vi "Read Folder.vi"(8 "error in (no error)":errorcluster, 11 "Context in":T1) -> (0 "error out":errorcluster, 3 "Context out":T1)   [LabVIEW 2020, in "DocTool.lvlib"]
uses:
  DocTool.lvlib
  TDefs/Context.ctl
  Events.ctl
  UserEvent.ctl
  TDefs/State.ctl
  TDefs/States.ctl
  TDefs/Single File Properties.ctl
  TDefs/FP Items Properties.ctl
  TDefs/FP Item Properties.ctl
  TDefs/CopyTag.ctl
  StateMachine.lvlib
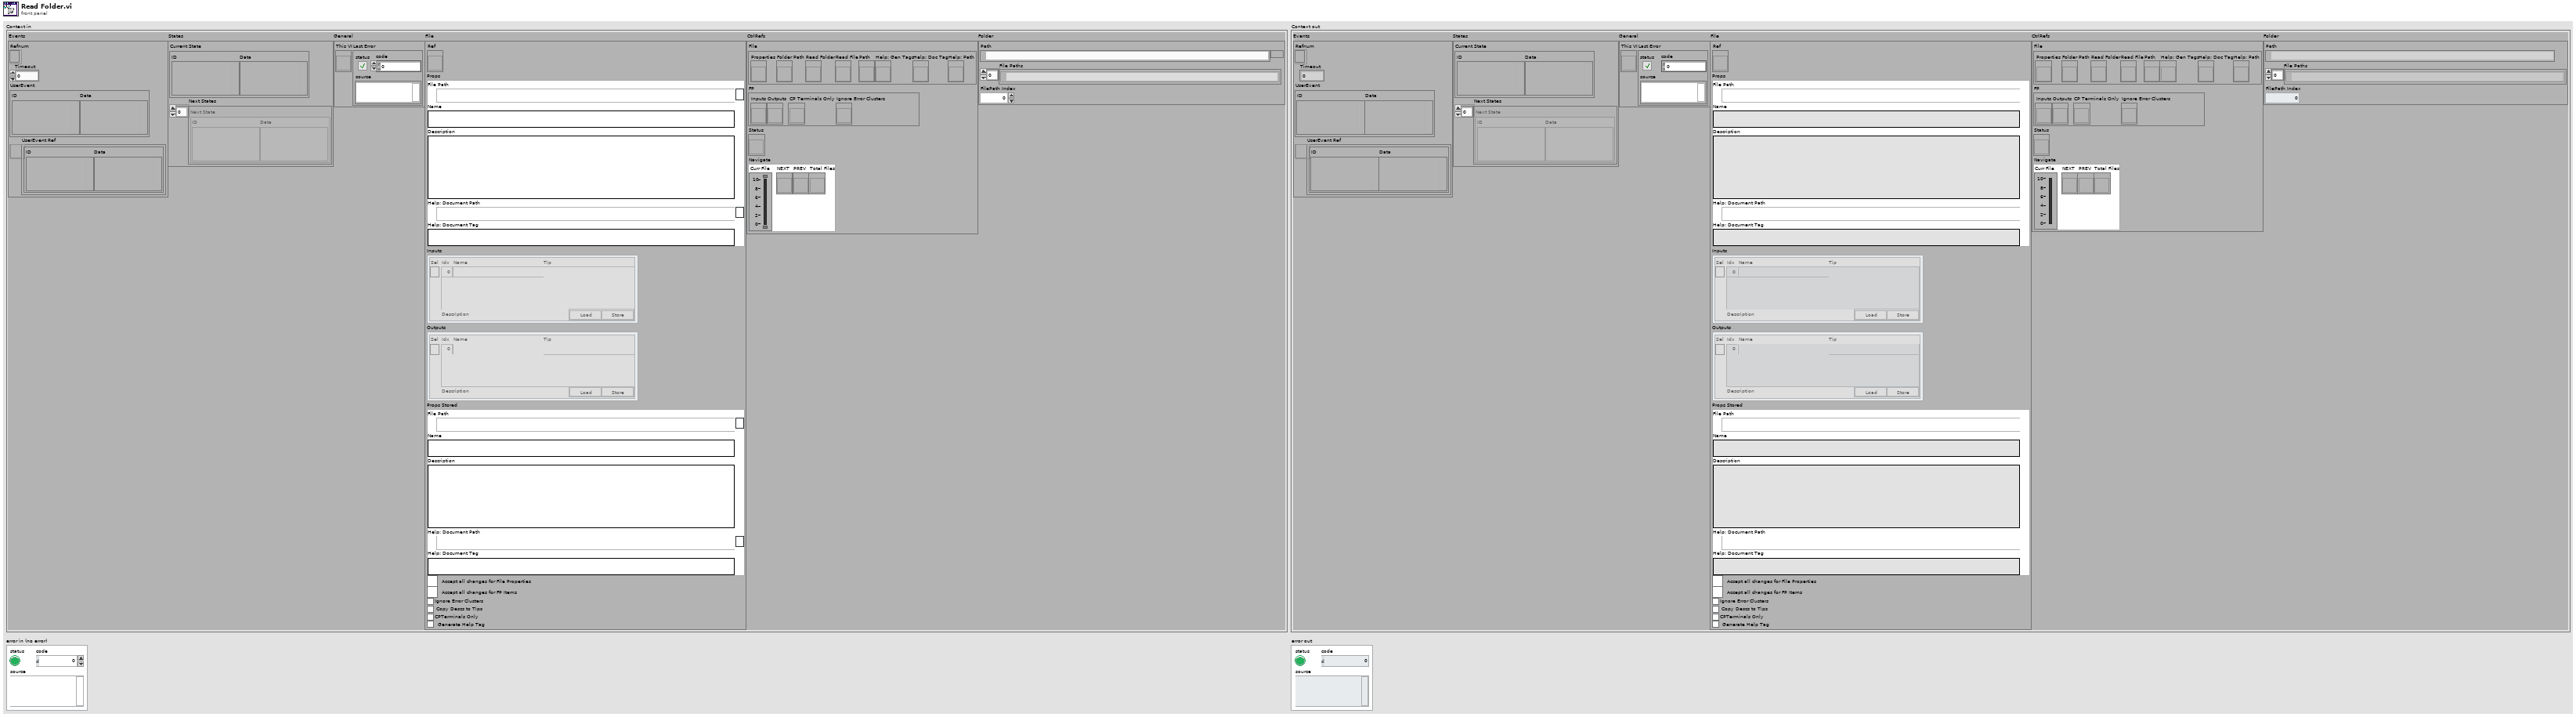
[diagram p1: front panel]
types:
  T1 = typedef "DocTool.lvlib/Context.ctl" = cluster{"Events":T2, "States":cluster{"Current State":T4, "Next States":T5}, "General":cluster{"This VI":refnum<vi>, "Last Error":errorcluster}, "File":cluster{"Ref":refnum<vi>, "Props":T6, "Inputs":T7, "Outputs":T7, "Props Stored":T6, "Write":bool, "Write FP":bool, "Ignore Error Clusters":bool, "Copy Descs to Tips":bool, "CPTerminals Only":bool, "Generate Help Tag":bool}, "CtrlRefs":cluster{"File":cluster{"Properties":refnum<vi>, "Folder Path":refnum<vi>, "Read Folder":refnum<vi>, "Read File":refnum<vi>, "Path":refnum<vi>, "Help: Gen Tags":refnum<vi>, "Help: Doc Tag":refnum<vi>, "Help: Path":refnum<vi>}, "FP":cluster{"Inputs":refnum<vi>, "Outputs":refnum<vi>, "CP Terminals Only":refnum<vi>, "Ignore Error Clusters":refnum<vi>}, "Status":refnum<vi>, "Navigate":cluster{"Curr File":refnum<vi>, "NEXT":refnum<vi>, "PREV":refnum<vi>, "Total Files":refnum<vi>}}, "Folder":cluster{"Path":path, "File Paths":path[], "FilePath Index":i32}}
  T2 = typedef "StateMachine.lvlib/Events.ctl" = cluster{"Refnum":refnum<event-registration>, "Timeout":i32, "UserEvent":T3, "UserEvent Ref":refnum<user-event>}
  T3 = typedef "StateMachine.lvlib/UserEvent.ctl" = cluster{"ID":variant, "Data":variant}
  T4 = typedef "StateMachine.lvlib/State.ctl" = cluster{"ID":variant, "Data":variant}
  T5 = typedef "StateMachine.lvlib/States.ctl" = T4[]
  T6 = typedef "DocTool.lvlib/Single File Properties.ctl" = cluster{"File Path":path, "Name":string, "Description":string, "Help: Document Path":path, "Help: Document Tag":string}
  T7 = typedef "DocTool.lvlib/FP Items Properties.ctl" = T8[]
  T8 = typedef "DocTool.lvlib/FP Item Properties.ctl" = cluster{"Sel":bool, "Idx":i32, "Name":string, "Description":string, "Tip":string, "Load Store":T9}
  T9 = typedef "DocTool.lvlib/CopyTag.ctl" = cluster{"Load":bool, "Store":bool}
  T10 = enum8{"Enabled", "Disabled", "Disabled and Grayed Out"}
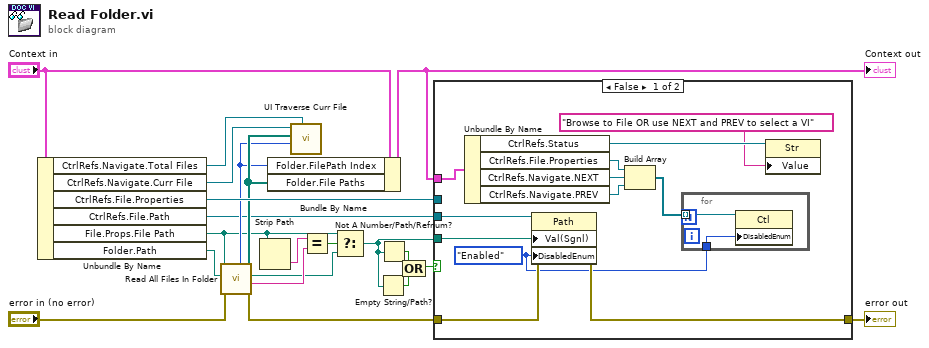
[diagram p0: block diagram]
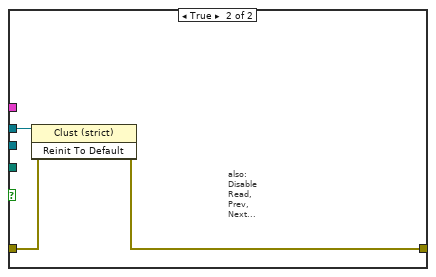
[diagram p2: hidden frame]
diagram:
  n1 = Unbundle By Name("Context in") -> ("CtrlRefs.Navigate.Total Files"=w19:refnum<vi>, "CtrlRefs.Navigate.Curr File"=w18:refnum<vi>, "CtrlRefs.File.Properties"=w20:refnum<vi>, "CtrlRefs.File.Path"=w6:refnum<vi>, "File.Props.File Path"=w11:path, "Folder.Path"=w5:path)
  n2 = call "Read All Files In Folder.vi"("error in (no error)"="error in (no error)", "FolderPath"=w5, "Old File Path"=w11) -> ("error out"=w21:errorcluster, "File Name"=w10:string, "New File Path"=w9:path, "File Paths"=w17:path[], "Index"=w16:i32)  [unwired: 4 in]
  n3 = Strip Path(path=w11) -> (name=w7:string)  [unwired: 1 out]
  n4 = Bundle By Name(cluster="Context in", "Folder.FilePath Index"=w16, "Folder.File Paths"=w17) -> (w1:T1)
  "Context out" <- w1
  n5 = call "UI Traverse Curr File.vi"("Tot Files"=w19, "Current File in"=w16, "File Paths"=w17, "Slide in"=w18) -> ()  [unwired: 7 in, 1 out]
  n6 = Equal?(x=w7, y=w10) -> (x = y?=w8:bool)
  n7 = Select(t=w11, s=w8, f=w9) -> (s? t:f=w12:path)
  n8 = Empty String/Path?(string/path=w12) -> (empty?=w13:bool)
  n9 = Not A Number/Path/Refnum?(number/path/refnum=w12) -> (NaN/Path/Refnum?=w14:bool)
  n10 = Compound Arithmetic op=OR(w14, w13) -> (w15:bool)
  n11 = case shown="False" w15 {
    tunnel: [w33 w36] -> w4
    tunnel: w21 -> [w32 w37]
    tunnel: w6 -> [w31 _]
    tunnel: w12 -> [w30 _]
    tunnel: w20 -> [_ w38]
    tunnel: w1 -> [w29 _]
    frame False {
      w28 = T10."Enabled" ("Disabled")
      n12 = Unbundle By Name(w29) -> ("CtrlRefs.Status"=w23:refnum<vi>, "CtrlRefs.File.Properties"=w24:refnum<vi>, "CtrlRefs.Navigate.NEXT"=w27:refnum<vi>, "CtrlRefs.Navigate.PREV"=w26:refnum<vi>)
      n13 = property on="Property Node" class="Path"(reference=w31, error in=w32, "Val(Sgnl)"=w30, "DisabledEnum"=w28) -> (error out=w33:errorcluster)  [unwired: 1 out]
      n14 = Build Array(w24, w27, w26) -> (w25:refnum<vi>[])
      n15 = for {
        tunnel: w28 -> [w35]
        tunnel: w25 -> [w34] mode=indexing
        n16 = property class="Ctl"(reference=w34, "DisabledEnum"=w35) -> ()  [unwired: 1 in, 2 out]
      }
      n17 = property class="Str"(reference=w23, "Value"="Browse to File OR use NEXT and PREV to select a VI") -> ()  [unwired: 1 in, 2 out]
    }
    frame True {
      # "also:\nDisable\nRead,\nPrev,\nNext..."
      n18 = invoke class="Clust (strict)" method="Reinit To Default"(reference=w38, error in=w37) -> (error out=w36:errorcluster)  [unwired: 1 in, 2 out]
    }
  }
  "error out" <- w4
